vi "wrapper_get_taskQueues.vi"(0 "HGF_ThreadWorker in":refnum<class "HGF_ThreadWorker.lvclass">, 2 "HGF_ThreadPool_Reference":refnum<class "HGF_Reference.lvclass">, 3 "timeout in ms (-1)":i32=-1, 5 "error in (no error)":errorcluster) -> (11 "got object?":bool, 14 "HGF_ThreadWorker out":refnum<class "HGF_ThreadWorker.lvclass">, 15 "taskQueue out":refnum<queue>, 16 "timeoutTaskQueueOut":i32, 17 "taskQueue in":refnum<queue>, 18 "timeoutTaskQueueIn":i32, 19 "error out":errorcluster)   [LabVIEW 2014, in "HGF_BaseClasses.lvlib" / "HGF_ThreadWorker.lvclass"]
uses:
  HGF_ThreadWorker.lvclass
  HGF_ThreadPool/HGF_ThreadPool.lvclass
  HGF_Reference/HGF_Reference.lvclass
  HGF_ThreadTask/HGF_ThreadTask.lvclass
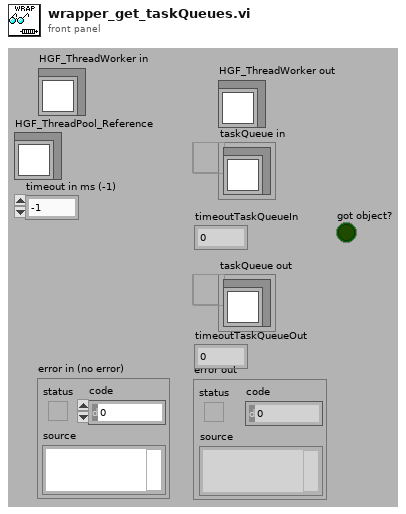
[diagram p1: front panel]
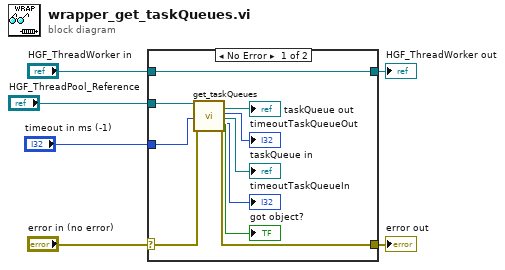
[diagram p0: block diagram]
diagram:
  n1 = case shown="No Error" "error in (no error)" {
    selector: "error in (no error)" -> [w13 w18]
    tunnel: [w12 w18] -> w5
    tunnel: [w16 w17] -> w3
    tunnel: "HGF_ThreadWorker in" -> [w16 w17]
    tunnel: "HGF_ThreadPool_Reference" -> [w15 _]
    tunnel: "timeout in ms (-1)" -> [w14 _]
    frame No Error {
      n2 = call "get_taskQueues.vi"("HGF_ThreadPool_Reference"=w15, "timeout in ms (-1)"=w14, "error in (no error)"=w13) -> ("got object?"=→"got object?":bool, "taskQueue out"=→"taskQueue out":refnum<queue>, "timeoutTaskQueueOut"=→"timeoutTaskQueueOut":i32, "taskQueue in"=→"taskQueue in":refnum<queue>, "timeoutTaskQueueIn"=→"timeoutTaskQueueIn":i32, "error out"=w12:errorcluster)  [unwired: 11 out]
    }
    frame Error {
    }
  }
  "error out" <- w5
  "HGF_ThreadWorker out" <- w3
